vi "Discretization_DiscretizeA.vi"(6 "dT_Seconds":dbl, 9 "ContA":T1, 11 "States":i32) -> (0 "Error":bool, 3 "DiscA":T1)   [LabVIEW 2019, in "Trajectory_Library.lvlib"]
doc: "Creates a new LINEAR SYSTEM data cluster with the specified values. \n\n\nInputs: \n - XXX -- XXX.\n\nOutputs:\n - XXX -- XXX."
uses:
  Trajectory_Library.lvlib
  <vilib>/Analysis/Matrix/Datatypes/RealMatrix.ctl
  MatBuilder_Create.vi
  <vilib>/Analysis/Matrix/Numeric/Multiply/Multiply - RM,R.vi
  <vilib>/Analysis/Matrix/NI_Matrix.lvlib
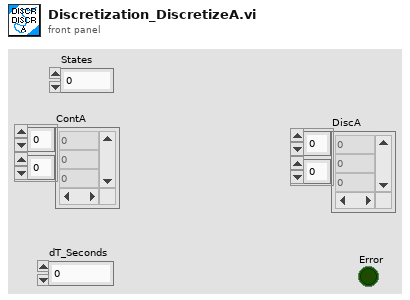
[diagram p1: front panel]
types:
  T1 = typedef "NI_Matrix.lvlib/RealMatrix.ctl" = dbl[][]
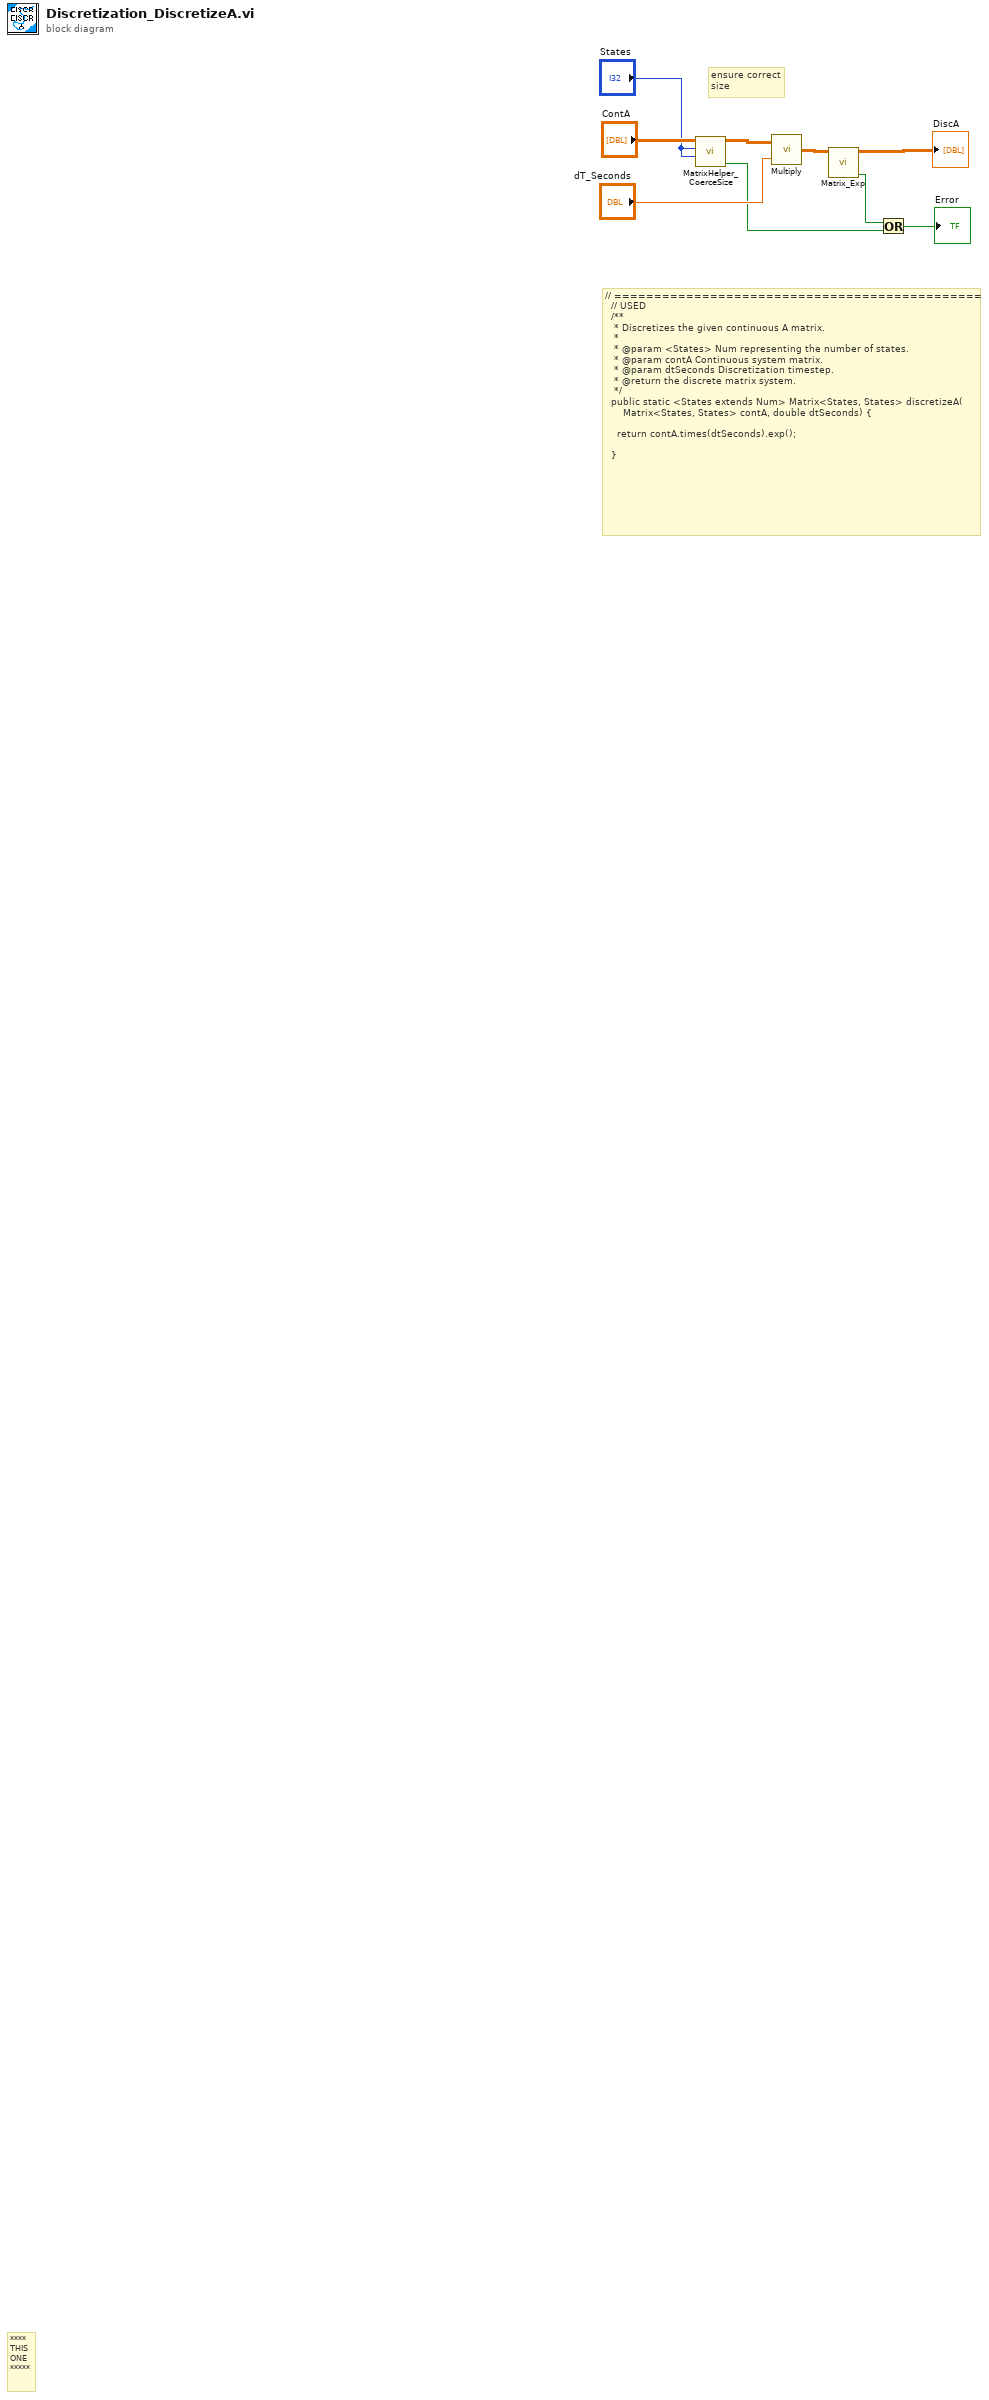
[diagram p0: block diagram]
diagram:
  # "// ==============================================\n  // USED\n  /**\n   * Discretizes the given continuous A matrix.\n   *\n   * @param <States> Num representing the number of states.\n   * @param contA Continuous system matrix.\n   * @param dtSeconds Discretization timestep.\n   * @return the discrete matrix system.\n   */\n  public static <States extends Num> Matrix<States, States> discretizeA(\n      Matrix<States, States> contA, double dtSeconds) {\n\n    return contA.times(dtSeconds).exp();\n\n  }"
  # "ensure correct\nsize"
  # "****\nTHIS\nONE\n*****"
  n1 = call "MatrixHelper_CoerceSize.vi"("Columns"="States", "Rows"="States", "input matrix"="ContA") -> ("Coerced"=w2:bool, "output matrix"=w7:T1)  [unwired: 7 in]
  n2 = call-poly <vilib>:"Multiply.vi"("Real Scalar c"="dT_Seconds", "Real Matrix A"=w7) -> ("A * c"=w5:T1)
  n3 = call "Matrix_Exp.vi"("input matrix"=w5) -> ("Error"=w3:bool, "output matrix"=→"DiscA":T1)  [unwired: 9 in]
  n4 = Or(x=w3, y=w2) -> (x .or. y?=→"Error":bool)
